vi "GoToAbsolutePosition(SubVI).vi"(6 "Absolute Volume Position in Syringe (in ul)":dbl, 7 "Volume of Syringe":dbl, 9 "Resolution of Pumping":T1(ring), 10 "Flow Rate (ul/min)":dbl, 11 "VISA Refnum in":refnum<visa-resource-name>) -> (3 "read buffer":string)   [LabVIEW 2020]
uses:
  <vilib>/Instr/_visa.llb/VISA Configure Serial Port (Instr).vi
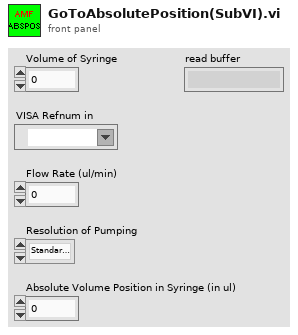
[diagram p1: front panel]
types:
  T1 = enum16{"Standard Pumping", "High Resolution Pumping"}
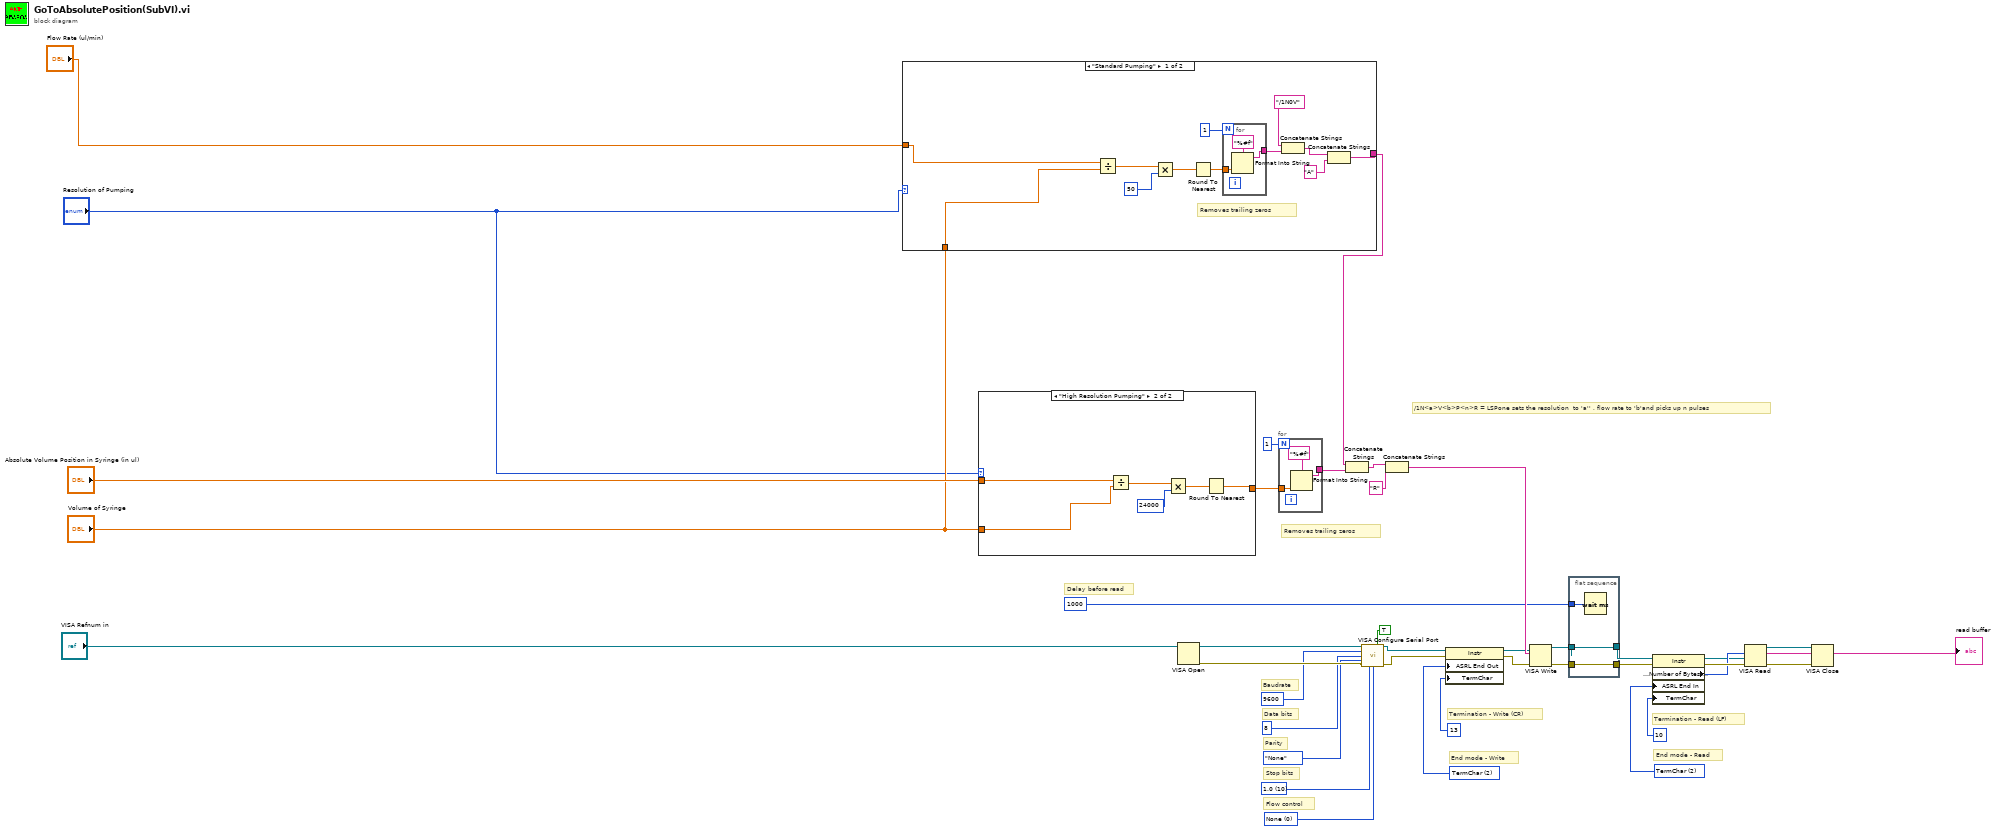
[diagram p0: block diagram]
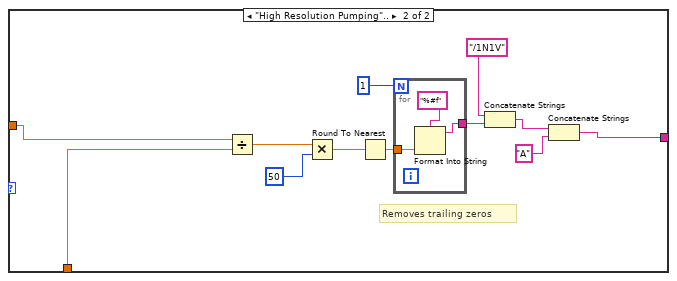
[diagram p2: hidden frame]
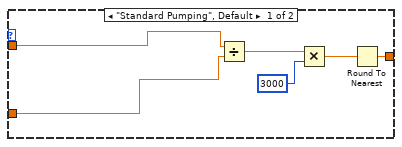
[diagram p3: hidden frame]
diagram:
  w3 = u16 2 items=["None", "Last Bit", "TermChar"] ("Serial Settings:End Mode for Reads")
  w6 = u16 2 items=["None", "Last Bit", "TermChar", "Break"] ("Serial Settings:End Mode for Writes")
  w7 = u16 0 items=["None", "XON/XOFF", "RTS/CTS", "XON/XOFF & RTS/CTS", "DTR/DSR", "XON/XOFF & DTR/DSR"] ("flow control (0:none)")
  w8 = u16 10 items=["1.0"=10, "1.5"=15, "2.0"=20] ("stop bits (10: 1 bit)")
  # "Removes trailing zeros"
  # "/1N<a>V<b>P<n>R = LSPone sets the resolution  to 'a'' , flow rate to 'b'and picks up n pulses"
  # "End mode - Read"
  # "Termination - Read (LF)"
  # "End mode - Write"
  # "Termination - Write (CR)"
  # "Flow control"
  # "Stop bits"
  # "Parity"
  # "Data bits"
  # "Baudrate"
  # "Delay before read"
  n1 = case shown="\"Standard Pumping\"" "Resolution of Pumping" {
    tunnel: [w44 w59] -> w33
    tunnel: "Volume of Syringe" -> [w41 w56]
    tunnel: "Flow Rate (ul/min)" -> [w40 w55]
    frame "Standard Pumping" {
      # "Removes trailing zeros"
      n2 = Divide(x=w40, y=w41) -> (x/y=w49:dbl)
      n3 = Multiply(x=w49, y=50) -> (x*y=w47:dbl)
      n4 = Round To Nearest(number=w47) -> (nearest integer value=w50:dbl)
      n5 = for {
        N: 1 -> [_]
        tunnel: w50 -> [w54]
        tunnel: [w53] -> w42
        n6 = Format Into String(format string="%#f", w54) -> (resulting string=w53:string)  [unwired: 2 in, 1 out]
      }
      n7 = Concatenate Strings("/1N0V", w42) -> (w46:string)
      n8 = Concatenate Strings(w46, "A") -> (w44:string)
    }
    frame "High Resolution Pumping".. {
      # "Removes trailing zeros"
      n9 = Divide(x=w55, y=w56) -> (x/y=w64:dbl)
      n10 = Multiply(x=w64, y=50) -> (x*y=w62:dbl)
      n11 = Round To Nearest(number=w62) -> (nearest integer value=w65:dbl)
      n12 = for {
        N: 1 -> [_]
        tunnel: w65 -> [w69]
        tunnel: [w68] -> w57
        n13 = Format Into String(format string="%#f", w69) -> (resulting string=w68:string)  [unwired: 2 in, 1 out]
      }
      n14 = Concatenate Strings("/1N1V", w57) -> (w61:string)
      n15 = Concatenate Strings(w61, "A") -> (w59:string)
    }
  }
  n16 = case shown="\"High Resolution Pumping\"" "Resolution of Pumping" {
    tunnel: [w75 w78] -> w31
    tunnel: "Volume of Syringe" -> [w71 w77]
    tunnel: "Absolute Volume Position in Syringe (in ul)" -> [w70 w76]
    frame "Standard Pumping", Default {
      n17 = Divide(x=w70, y=w71) -> (x/y=w74:dbl)
      n18 = Multiply(x=w74, y=3000) -> (x*y=w72:dbl)
      n19 = Round To Nearest(number=w72) -> (nearest integer value=w75:dbl)
    }
    frame "High Resolution Pumping" {
      n20 = Divide(x=w76, y=w77) -> (x/y=w81:dbl)
      n21 = Multiply(x=w81, y=24000) -> (x*y=w79:dbl)
      n22 = Round To Nearest(number=w79) -> (nearest integer value=w78:dbl)
    }
  }
  n23 = VISA Open(VISA resource name="VISA Refnum in") -> (VISA resource name=w15:refnum<visa-resource-name>, error out=w14:errorcluster)  [unwired: 4 in]
  n24 = for {
    N: 1 -> [_]
    tunnel: w31 -> [w84]
    tunnel: [w83] -> w32
    n25 = Format Into String(format string="%#f", w84) -> (resulting string=w83:string)  [unwired: 2 in, 1 out]
  }
  n26 = Concatenate Strings(w33, w32) -> (w29:string)
  n27 = call-poly "VISA Configure Serial Port"("VISA resource name"=w15, "Enable Termination\nChar (T)"=TRUE, "baud rate (9600)"=u32 9600, "data bits (8)"=u16 8, "parity (0:none)"=enum16{"None", "Odd", "Even", "Mark", "Space"}."None", "error in (no error)"=w14, "stop bits (10: 1 bit)"=w8, "flow control (0:none)"=w7) -> ("VISA resource name out"=w22:refnum<visa-resource-name>, "error out"=w21:errorcluster)  [unwired: 1 in, 5 out]
  n28 = Concatenate Strings(w29, "R") -> (w34:string)
  n29 = property class="Instr"(reference=w22, error in=w21, "ASRL End Out"=w6, "TermChar"=u8 13 ("Message Based Settings:Termination Character")) -> (reference out=w20:refnum<visa-resource-name>, error out=w19:errorcluster)
  n30 = VISA Write(VISA resource name=w20, write buffer=w34, error in (no error)=w19) -> (VISA resource name out=w26:refnum<visa-resource-name>, error out=w28:errorcluster)  [unwired: 1 out]
  n31 = flat-sequence {
    tunnel: w28 -> [w86]
    tunnel: [w86] -> w27
    tunnel: w26 -> [w85]
    tunnel: [w85] -> w12
    tunnel: u32 1000 ("delay before read (ms)") -> [w87]
    frame #0 {
      n32 = Wait (ms)(milliseconds to wait=w87) -> ()  [unwired: 1 out]
    }
  }
  n33 = property class="Instr"(reference=w12, error in=w27, "ASRL End In"=w3, "TermChar"=u8 10 ("Message Based Settings:Termination Character")) -> (reference out=w13:refnum<visa-resource-name>, error out=w24:errorcluster, "Serial Settings:Number of Bytes at Serial Port"=w23:u32)
  n34 = VISA Read(VISA resource name=w13, byte count=w23, error in (no error)=w24) -> (VISA resource name out=w17:refnum<visa-resource-name>, read buffer=→"read buffer":string, error out=w16:errorcluster)  [unwired: 1 out]
  n35 = VISA Close(VISA resource name=w17, error in (no error)=w16) -> ()  [unwired: 1 out]
